vi "_Main.vi"   [LabVIEW 2017, in "Claw.lvlib"]
uses:
  Claw.lvlib
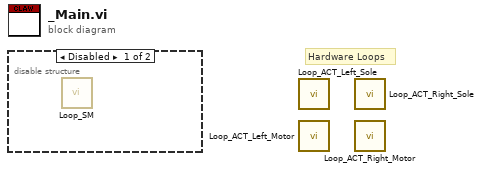
[diagram p0: block diagram]
diagram:
  # "Hardware Loops"
  n1 = disable-structure shown="Disabled" {
    frame Disabled {
      n2 = call "Loop_SM.vi"() -> ()  [unwired: 12 in]
    }
    frame Enabled {
    }
  }
  n3 = call "Loop_ACT_Left_Sole.vi"() -> ()  [unwired: 12 in]
  n4 = call "Loop_ACT_Left_Motor.vi"() -> ()  [unwired: 12 in]
  n5 = call "Loop_ACT_Right_Sole.vi"() -> ()  [unwired: 12 in]
  n6 = call "Loop_ACT_Right_Motor.vi"() -> ()  [unwired: 12 in]
